vi "TestTabDisabled.vi"() -> ()   [LabVIEW 2022 SP3]
uses:
  Classes/TopLevel/Typedefs/PurgeMode--Enum.ctl
  Classes/TopLevel/Typedefs/AdvPrinterControl--Tabs.ctl
panel:
  in  "OK":bool
  in  "PrinterControls":T1
  out "ImageMain":T2(plugin-control)
  in  "Head6 Temp 1":string
  in  "Head5 Temp 1":string
  in  "Head4 Temp 1":string
  in  "Head3 Temp 1":string
  in  "Head2 Temp 1":string
  in  "Jog (+) 1":bool
  in  "Jog (-) 1":bool
  in  "Mode H1":T3
  in  "Mode H2":T3
  in  "Mode H3":T3
  in  "Mode H4":T3
  in  "Mode H5":T3
  in  "Mode H6":T3
  in  "Prime Repeats1 1":u8=1 min=1
  in  "Prime Repeats1 2":u8=1
  in  "Prime Repeats1 3":u8=1
  in  "Prime Repeats1 4":u8=1
  in  "Prime Repeats1 5":u8=1
  in  "Prime Repeats1 6":u8=1
  in  "StartPrime1 6":bool
  in  "StartPrime1 5":bool
  in  "StartPrime1 4":bool
  in  "StartPrime1 3":bool
  in  "StartPrime1 2":bool
  in  "StartPrime1 1":bool
  in  "Head1 Temp 1":string
  in  "Stage Head6":bool
  in  "Stage Head5":bool
  in  "Stage Head4":bool
  in  "Stage Head3":bool
  in  "Stage Head2":bool
  in  "Stage Head1":bool
  in  "Jog (+) 2":bool
  in  "Jog (-) 2":bool
  in  "Stage Recipe XML File Path":path
  in  "Start":bool
  in  "Stage Move Status":i32(listbox)
  in  "Idle Intervals (s)":dbl=0.1
  in  "IdlePrint":bool
  # "Jogging"
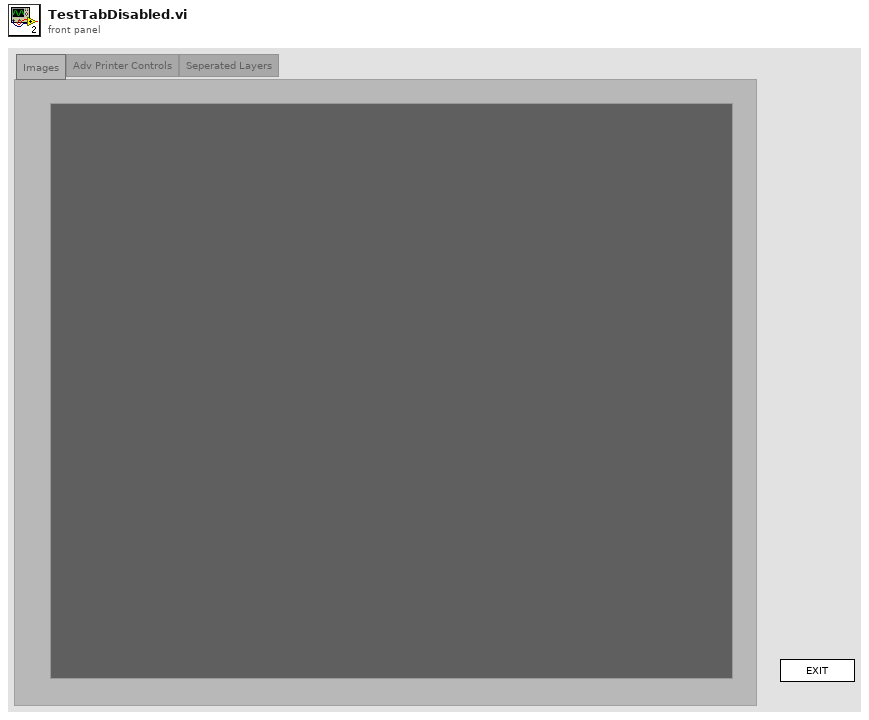
[diagram p1: front panel]
types:
  T1 = typedef "AdvPrinterControl--Tabs.ctl" = enum32{"Images", "Adv Printer Controls", "Seperated Layers"}
  T2 = typedef "IMAQ Image.ctl" = refnum<image>
  T3 = typedef "PurgeMode--Enum.ctl" = enum16{"Pre-Purge", "Purge", "Spit", "Prime"}
  T4 = enum8{"Enabled", "Disabled", "Disabled and Grayed Out"}
  T5 = enum32{"Invalid", "Standard", "Closed", "Hidden", "Minimized", "Maximized"}
  T6 = enum32{"invalid app kind", "Development System", "Run Time System", "Student Edition", "Embedded LabVIEW", "Evaluation", "Custom"}
  T7 = cluster{"Core":cluster{"Current VI Reference":refnum<vi>, "Close Panel on Exit?":bool}, "Your Boolean data":bool, "Your string data":string}
  T8 = cluster{"Current VI Reference":refnum<vi>, "Close Panel on Exit?":bool}
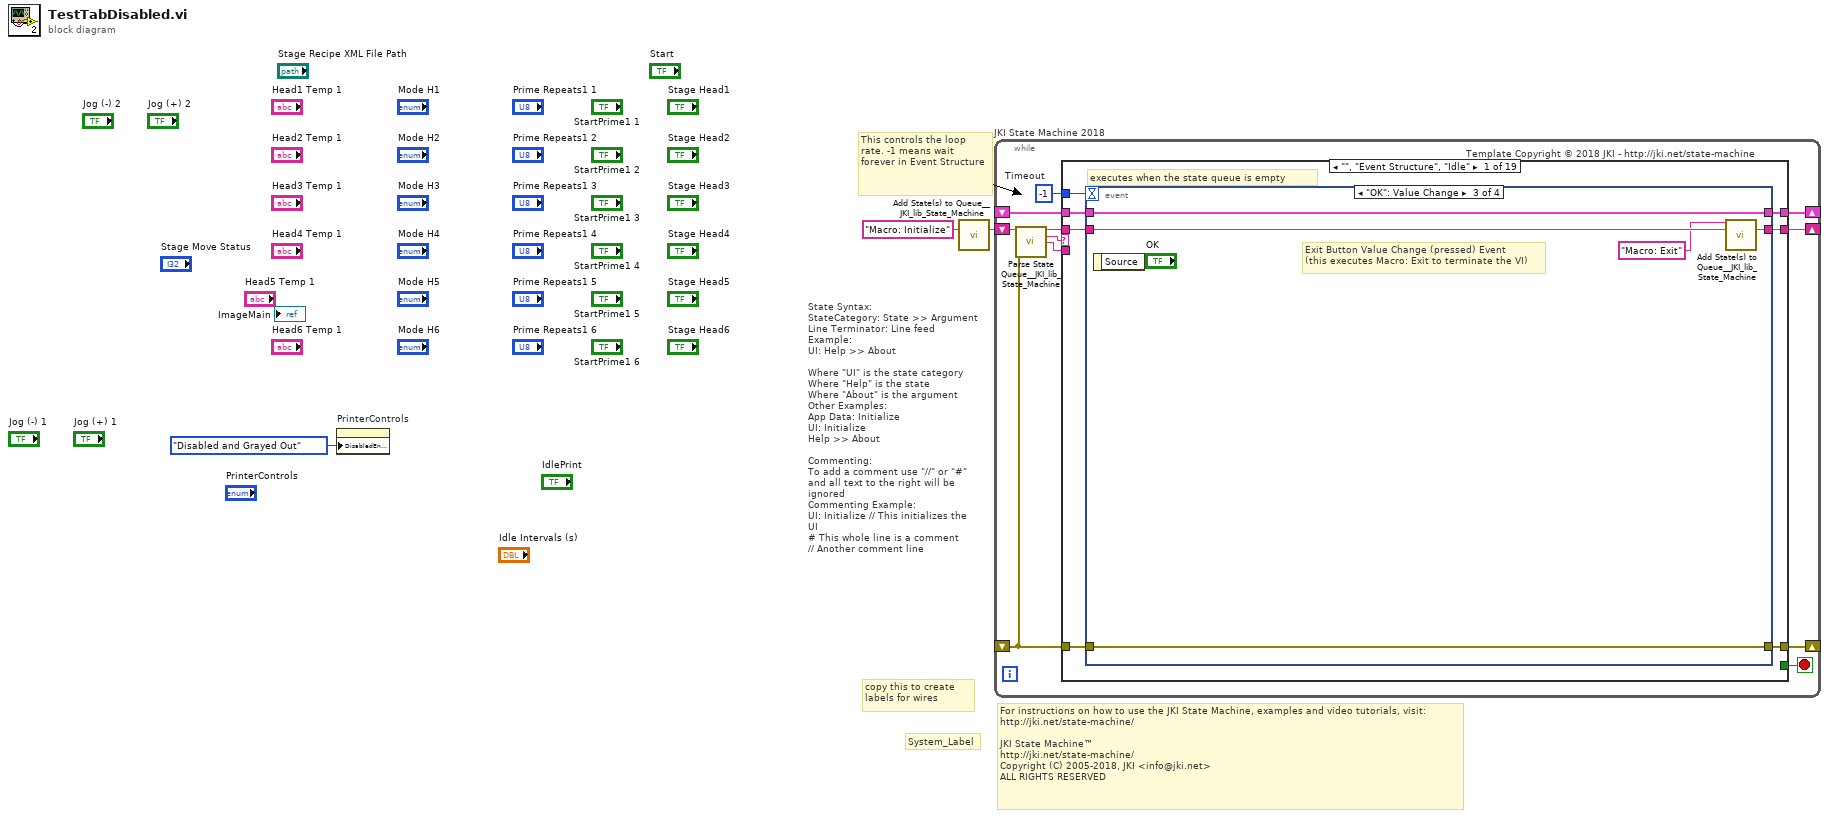
[diagram p0: block diagram]
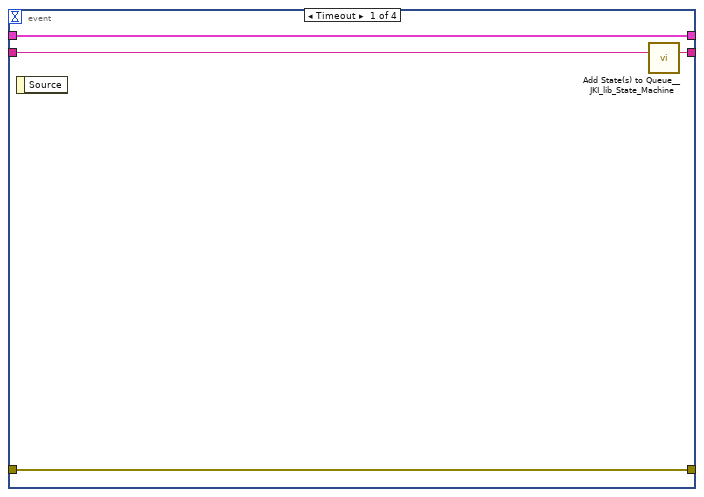
[diagram p2: hidden frame]
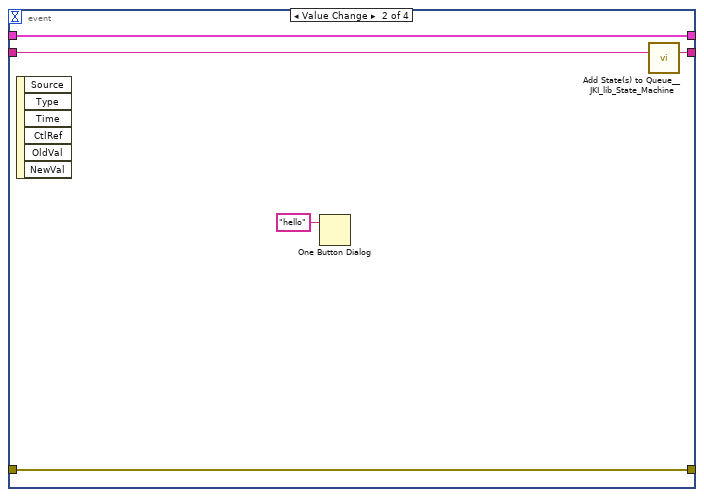
[diagram p3: hidden frame]
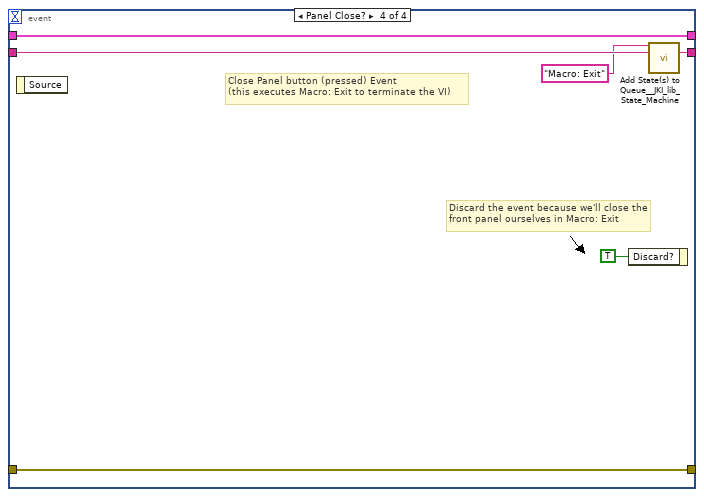
[diagram p4: hidden frame]
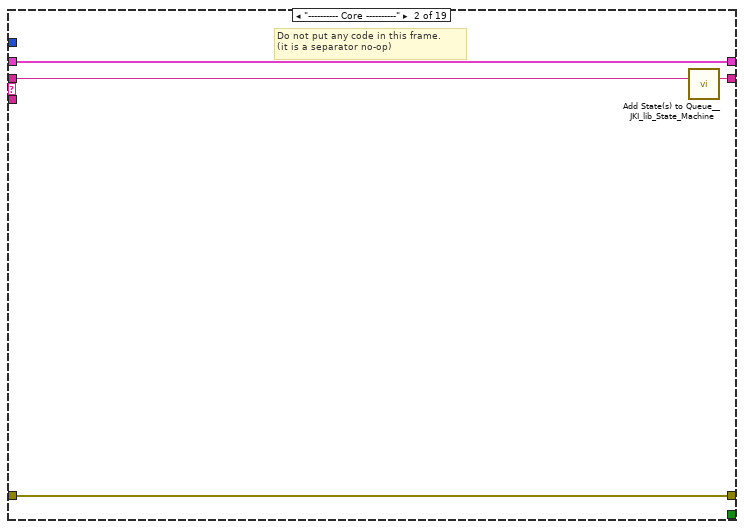
[diagram p5: hidden frame]
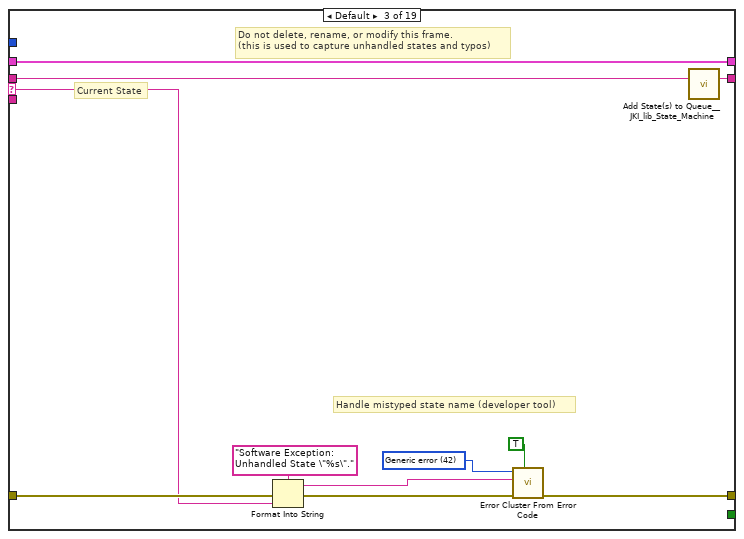
[diagram p6: hidden frame]
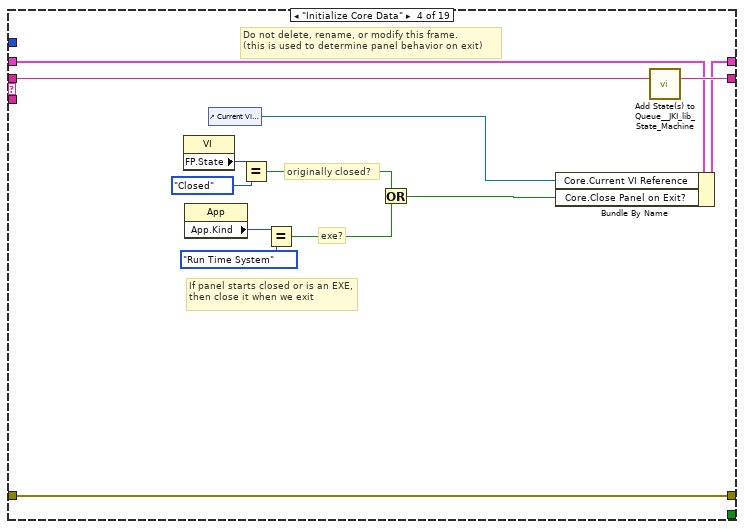
[diagram p7: hidden frame]
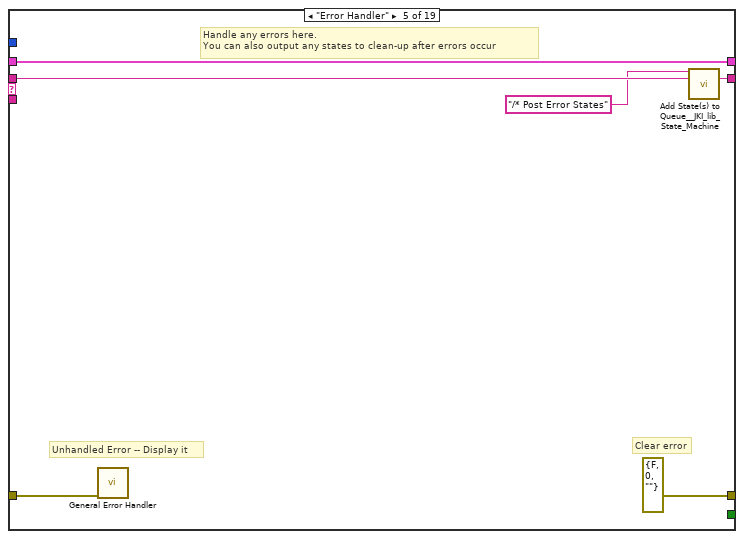
[diagram p8: hidden frame]
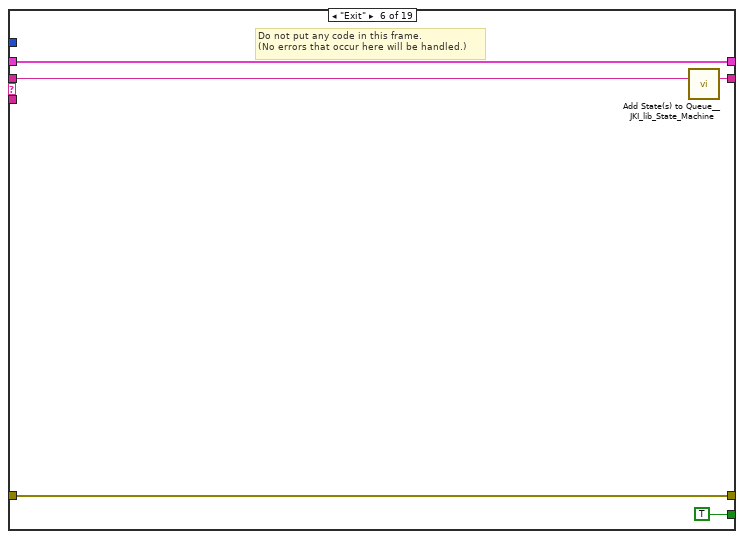
[diagram p9: hidden frame]
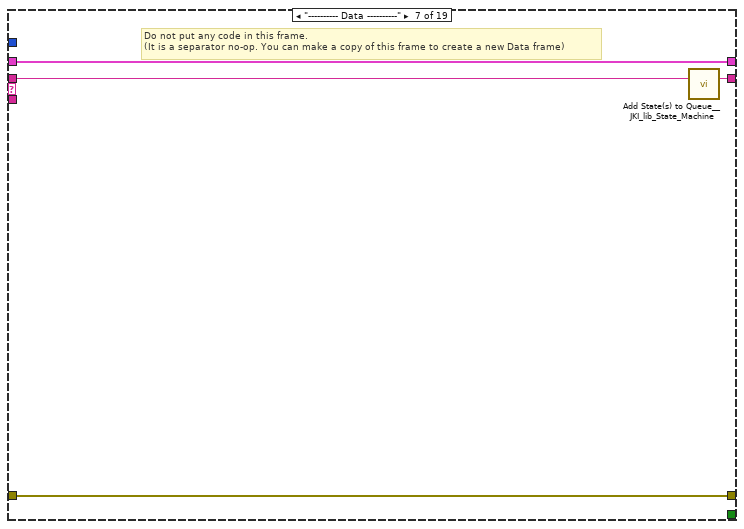
[diagram p10: hidden frame]
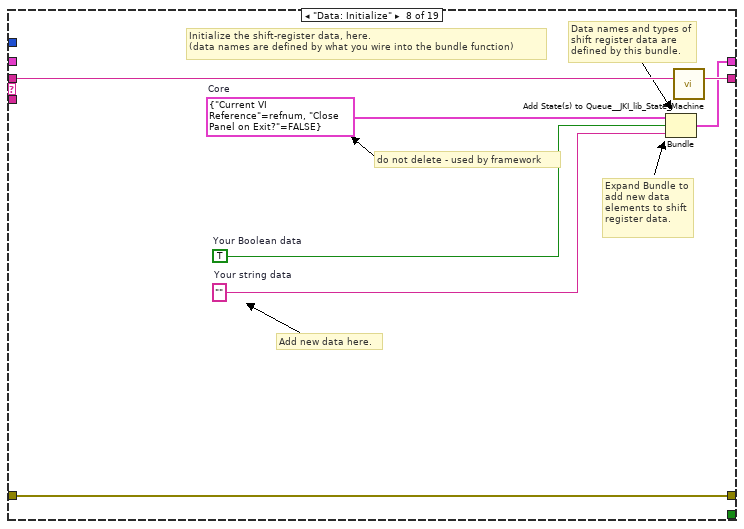
[diagram p11: hidden frame]
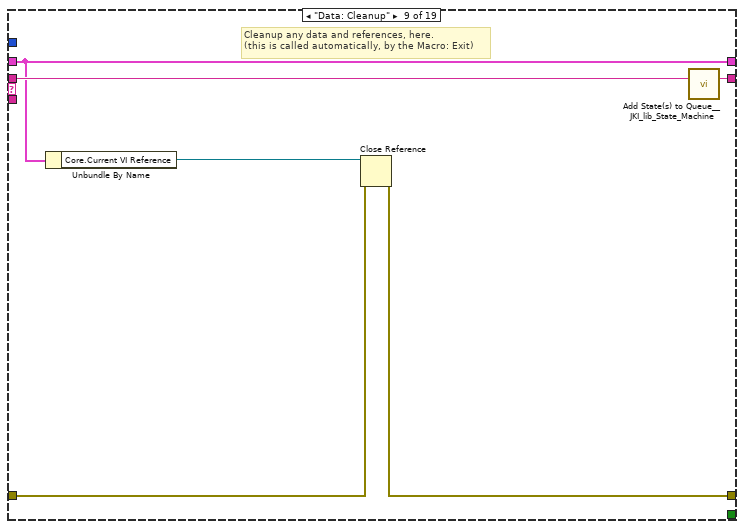
[diagram p12: hidden frame]
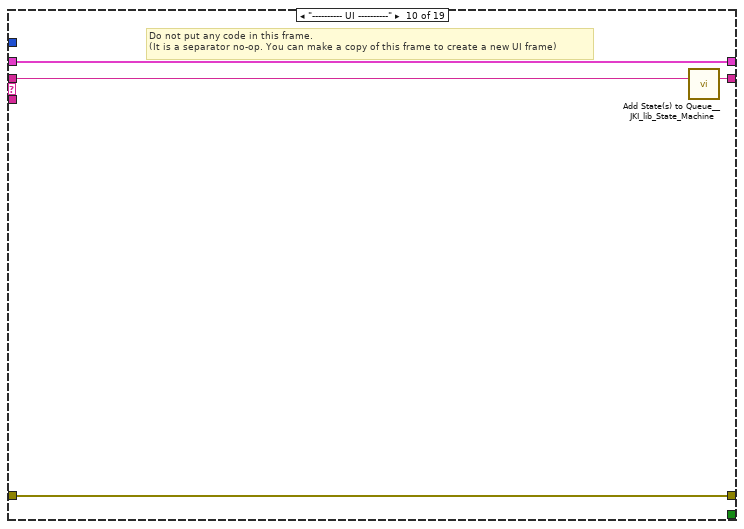
[diagram p13: hidden frame]
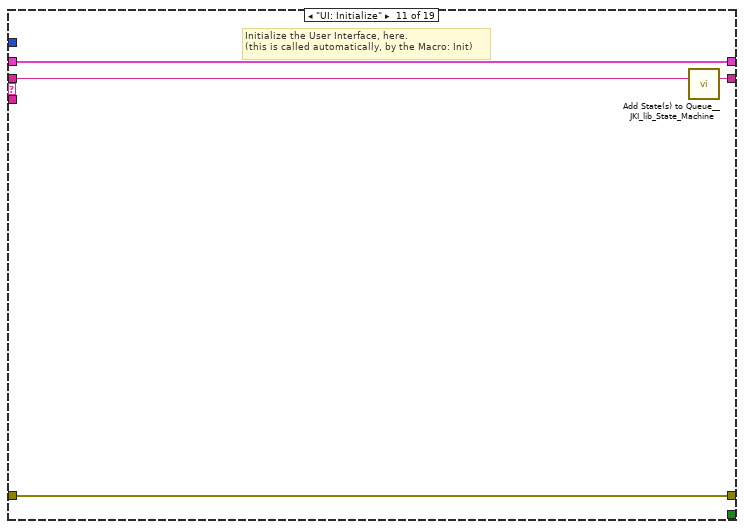
[diagram p14: hidden frame]
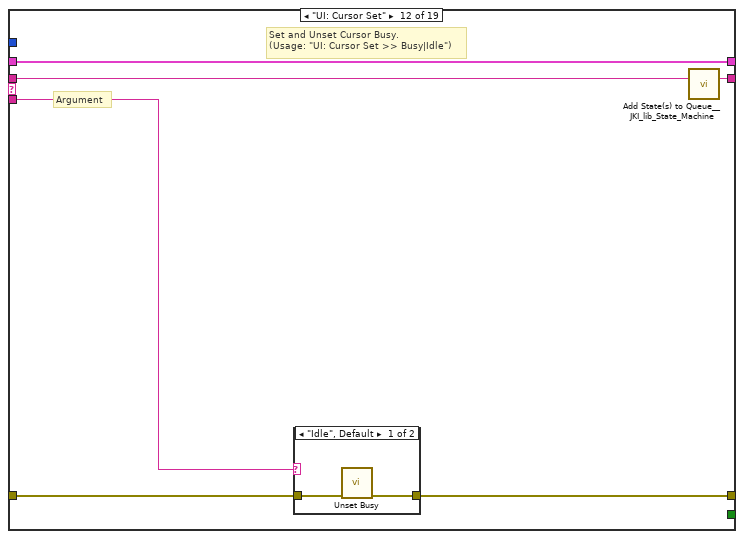
[diagram p15: hidden frame]
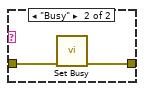
[diagram p16: hidden frame]
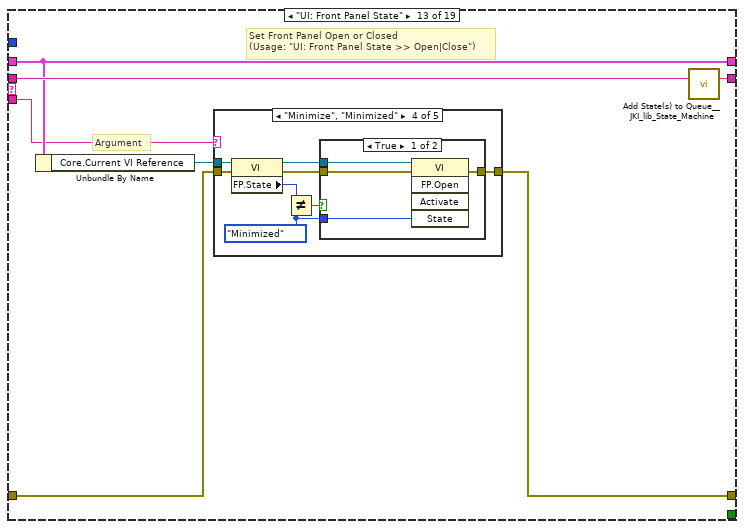
[diagram p17: hidden frame]
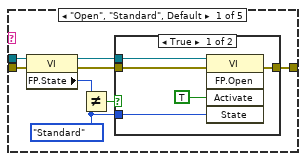
[diagram p18: hidden frame]
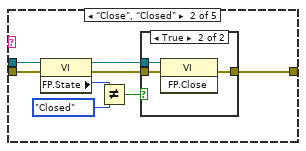
[diagram p20: hidden frame]
diagram:
  # "For instructions on how to use the JKI State Machine, examples and video tutorials, visit:\nhttp://jki.net/state-machine/\n\nJKI State Machine™\nhttp://jki.net/state-machine/\nCopyright (C) 2005-2018, JKI <info@jki.net>\nALL RIGHTS RESERVED"
  # "State Syntax:\nStateCategory: State >> Argument\nLine Terminator: Line feed\nExample:\nUI: Help >> About\n\nWhere \"UI\" is the state category\nWhere \"Help\" is the state\nWhere \"About\" is the argument\nOther Examples:\nApp Data: Initialize\nUI: Initialize\nHelp >> About\n\nCommenting:\nTo add a comment use \"//\" or \"#\" and all text to the right will be ignored\nCommenting Example:\nUI: Initialize // This initializes the UI\n# This whole line is a comment\n// Another comment line"
  # "copy this to create labels for wires"
  # "This controls the loop rate. -1 means wait forever in Event Structure"
  # "System_Label"
  n1 = property on="PrinterControls" class="TabCtl (strict)"("DisabledEnum"=T4."Disabled and Grayed Out" ("Disabled")) -> ()  [unwired: 2 in, 2 out]
  n2 = call <vilib>:"Add State(s) to Queue__JKI_lib_State_Machine.vi"("State(s) in (\"\")"="Macro: Initialize") -> ("States Out"=w2:string)  [unwired: 14 in]
  n3 = while "JKI State Machine 2018" {
    shift-right: [w7] -> _
    shift-left: _ -> [w6]
    shift-right: [w10] -> _
    shift-left: _ -> [w4]
    shift-right: [w9] -> _
    shift-left: w2 -> [w11]
    stop <- w8 stop-if-true
    w5 = -1  # Timeout
    # "Template Copyright © 2018 JKI - http://jki.net/state-machine"
    n4 = call <vilib>:"Parse State Queue__JKI_lib_State_Machine.vi"("State Queue"=w11, "Error In (no error)"=w4) -> ("Remaining States"=w13:string, "Current State"=w14:string, "Arguments"=w12:string)  [unwired: 11 in]
    n5 = case shown="\"\", \"Event Structure\", \"Idle\"" w14 {
      selector: w14 -> [_ _ w46 _ _ _ _ _ _ _ _ _ _ _ _ _ _ _ _]
      tunnel: w13 -> [w21 w45 w50 w69 w75 w80 w84 w91 w97 w101 w105 w111 w122 w191 w196 w206 w210 w214 w218]
      tunnel: w12 -> [_ _ _ _ _ _ _ _ _ _ _ w106 w116 _ _ _ _ _ _]
      tunnel: w6 -> [w19 w42 w48 w62 w72 w78 w81 _ w92 w98 w103 w109 w118 w188 w193 w203 w207 w211 w215]
      tunnel: [w18 w43 w52 w66 errorcluster {"status"=FALSE, "code"=0, "source"=""} ("error out") w77 w82 w88 w93 w99 w102 w107 w119 w189 w194 w204 w208 w212 w216] -> w10
      tunnel: w4 -> [w17 w43 w51 w66 w71 w77 w82 w88 w94 w99 w102 w108 w120 w189 w194 w204 w208 w212 w216]
      tunnel: [w20 w44 w49 w68 w74 w79 w83 w90 w96 w100 w104 w110 w121 w190 w195 w205 w209 w213 w217] -> w9
      tunnel: [_ _ _ _ _ TRUE _ _ _ _ _ _ _ _ _ _ _ _ _] -> w8
      tunnel: [w16 w42 w48 w67 w72 w78 w81 w89 w92 w98 w103 w109 w118 w188 w193 w203 w207 w211 w215] -> w7
      tunnel: w5 -> [w15 _ _ _ _ _ _ _ _ _ _ _ _ _ _ _ _ _ _]
      frame "", "Event Structure", "Idle" {
        # "executes when the state queue is empty"
        n6 = event shown="[2] \"OK\": Value Change" {
          selector: _ -> [_ _ _ _]
          dyn-events: _ -> [_ _ _ _]
          timeout: w15 -> [_ _ _ _]
          tunnel: w21 -> [w25 w30 w35 w41]
          tunnel: [w24 w29 w34 w40] -> w20
          tunnel: w19 -> [w22 w27 w32 w38]
          tunnel: [w23 w28 w33 w39] -> w18
          tunnel: w17 -> [w23 w28 w33 w39]
          tunnel: [w22 w27 w32 w38] -> w16
          event Timeout {
            n7 = event-data() -> ()  [unwired: 1 in, 1 out]
            n8 = call <vilib>:"Add State(s) to Queue__JKI_lib_State_Machine.vi"("State(s) in (\"\")"=w25) -> ("States Out"=w24:string)  [unwired: 14 in]
          }
          event Value Change {
            n9 = event-data() -> ()  [unwired: 1 in, 6 out]
            n10 = One Button Dialog(message="hello") -> ()  [unwired: 1 in, 1 out]
            n11 = call <vilib>:"Add State(s) to Queue__JKI_lib_State_Machine.vi"("State(s) in (\"\")"=w30) -> ("States Out"=w29:string)  [unwired: 14 in]
          }
          event "OK": Value Change {
            # "Exit Button Value Change (pressed) Event\n(this executes Macro: Exit to terminate the VI)"
            n12 = event-data() -> ()  [unwired: 1 in, 1 out]
            n13 = call <vilib>:"Add State(s) to Queue__JKI_lib_State_Machine.vi"("State(s) in Front (\"\")"="Macro: Exit", "State(s) in (\"\")"=w35) -> ("States Out"=w34:string)  [unwired: 13 in]
          }
          event Panel Close? {
            # "Discard the event because we'll close the front panel ourselves in Macro: Exit"
            # "Close Panel button (pressed) Event\n(this executes Macro: Exit to terminate the VI)"
            n14 = event-data() -> ()  [unwired: 1 in, 1 out]
            n15 = event-data("Discard?"=TRUE) -> ()  [unwired: 1 in, 1 out]
            n16 = call <vilib>:"Add State(s) to Queue__JKI_lib_State_Machine.vi"("State(s) in Front (\"\")"="Macro: Exit", "State(s) in (\"\")"=w41) -> ("States Out"=w40:string)  [unwired: 13 in]
          }
        }
      }
      frame "---------- Core ----------" {
        # "Do not put any code in this frame.\n(it is a separator no-op)"
        n17 = call <vilib>:"Add State(s) to Queue__JKI_lib_State_Machine.vi"("State(s) in (\"\")"=w45) -> ("States Out"=w44:string)  [unwired: 14 in]
      }
      frame Default {
        w55 = 42 items=["No error", "Argument error", "Memory is full", "Out of zone", "End of file", "File already open", "Generic file I/O error", "File not found", "File permission error", "Disk is full", "Duplicate path", "Too many files open", "System feature not enabled", "Resource file not found", "Cannot add resource", "Resource not found", "Image not found", "Image memory error", "Pen does not exist", "Config type invalid", "Config token not found", "Config parse error", "Config memory error", "Bad external code format", "Bad external code offset", "External code not present", "Null window", "Destroy window error", "Null menu", "Print aborted", "Bad print record", "Print driver error", "Windows error during printing", "Memory error during printing", "Print dialog error", "Generic print error", "Invalid device refnum", "Device not found", "Device parameter error", "Device unit error", "Cannot open device", "Device call aborted", "Generic error", "Cancelled by user", "Object ID too low", "Object ID too high", "Object not in heap", "Unknown heap", "Unknown object (invalid DefProc)", "Unknown object (DefProc not in table)", "Message out of range", "Invalid (null) method", "Unknown message", "Manager call not supported", "Bad address", "Network operation in progress", "Network operation timed out", "Connection is busy", "Network attribute not supported", "Network error", "Address in use", "System out of memory", "Connection aborted", "Connection refused", "Not connected", "Already connected", "Connection closed", "Initialization error (interapplication manager)", "Bad occurrence", "Wait on unbound occurrence handler", "Occurrence queue overflow", "Datalog type conflict", "Unused", "Unrecognized type (interapplication manager)", "Memory corrupt", "Failed to make temporary DLL", "Old CIN version", "Drag socket not found", "Failed to load drop-object", "Failed to register OLE object", "Failed to release OLE object", "Format specifier type mismatch", "Unknown format specifier", "Too few format specifiers", "Too many format specifiers", "Scan failed", "Newer CIN version", "Error converting to variant", "Runtime menu error", "Password tampered", "Variant attribute not found", "Incompatible variant data type", "Event data is not available", "Event Store is not present", "Occurrence is not found", "Event Queue is not created", "Event info is not available", "Refnum passed is NULL", "Error retrieving Class GUID", "Error retrieving CoClass GUID", "Error retrieving TypeLib GUID.", "Bad built application magic bytes.", "Specific driver is different from the specific driver associated with the Logical Name.", "There is no session opened to the class driver.", "Max Error", "MAX - Error with config objects", "MAX - Error loading configuration", "MAX - Group not supported"]
        # "Current State"
        # "Do not delete, rename, or modify this frame.\n(this is used to capture unhandled states and typos)"
        # "Handle mistyped state name (developer tool)"
        n18 = Format Into String(format string="Software Exception: Unhandled State \"%s\"." ("message"), error in=w51, w46) -> (resulting string=w54:string, error out=w53:errorcluster)  [unwired: 1 in]
        n19 = call <vilib>:"Error Cluster From Error Code.vi"("show call chain? (False)"=TRUE, "error in (no error)"=w53, "error message (\"\")"=w54, "error code (0)"=w55) -> ("error out"=w52:errorcluster)  [unwired: 5 in]
        n20 = call <vilib>:"Add State(s) to Queue__JKI_lib_State_Machine.vi"("State(s) in (\"\")"=w50) -> ("States Out"=w49:string)  [unwired: 14 in]
      }
      frame "Initialize Core Data" {
        # "Do not delete, rename, or modify this frame.\n(this is used to determine panel behavior on exit)"
        # "originally closed?"
        # "exe?"
        # "If panel starts closed or is an EXE, then close it when we exit"
        n21 = property class="VI"() -> ("FP.State"=w59:T5)  [unwired: 2 in, 2 out]
        n22 = property class="App"() -> ("App.Kind"=w65:T6)  [unwired: 2 in, 2 out]
        n23 = control-ref of="Current VI Reference"() -> (w60:refnum<vi>)
        n24 = Equal?(x=w59, y=T5."Closed" ("Front Panel Window:State")) -> (x = y?=w57:bool)
        n25 = Equal?(x=w65, y=T6."Run Time System" ("Application:Kind")) -> (x = y?=w63:bool)
        n26 = Or(x=w57, y=w63) -> (x .or. y?=w61:bool)
        n27 = Bundle By Name(cluster=w62, "Core.Current VI Reference"=w60, "Core.Close Panel on Exit?"=w61) -> (w67:T7)
        n28 = call <vilib>:"Add State(s) to Queue__JKI_lib_State_Machine.vi"("State(s) in (\"\")"=w69) -> ("States Out"=w68:string)  [unwired: 14 in]
      }
      frame "Error Handler" {
        # "Unhandled Error -- Display it"
        # "Handle any errors here.\nYou can also output any states to clean-up after errors occur"
        # "Clear error"
        n29 = call <vilib>:"General Error Handler.vi"("error in (no error)"=w71) -> ()  [unwired: 10 in, 5 out]
        n30 = call <vilib>:"Add State(s) to Queue__JKI_lib_State_Machine.vi"("State(s) in Front (\"\")"="/* Post Error States", "State(s) in (\"\")"=w75) -> ("States Out"=w74:string)  [unwired: 13 in]
      }
      frame "Exit" {
        # "Do not put any code in this frame.\n(No errors that occur here will be handled.)"
        n31 = call <vilib>:"Add State(s) to Queue__JKI_lib_State_Machine.vi"("State(s) in (\"\")"=w80) -> ("States Out"=w79:string)  [unwired: 14 in]
      }
      frame "---------- Data ----------" {
        # "Do not put any code in this frame.\n(It is a separator no-op. You can make a copy of this frame to create a new Data frame)"
        n32 = call <vilib>:"Add State(s) to Queue__JKI_lib_State_Machine.vi"("State(s) in (\"\")"=w84) -> ("States Out"=w83:string)  [unwired: 14 in]
      }
      frame "Data: Initialize" {
        w85 = T8 {"Current VI Reference"=refnum, "Close Panel on Exit?"=FALSE}  # Core
        w87 = TRUE  # Your Boolean data
        w86 = ""  # Your string data
        # "do not delete - used by framework"
        # "Expand Bundle to add new data elements to shift register data."
        # "Add new data here."
        # "Data names and types of shift register data are defined by this bundle."
        # "Initialize the shift-register data, here.\n(data names are defined by what you wire into the bundle function)"
        n33 = Bundle("Core"=w85, "Your Boolean data"=w87, "Your string data"=w86) -> (w89:T7)  [unwired: 1 in]
        n34 = call <vilib>:"Add State(s) to Queue__JKI_lib_State_Machine.vi"("State(s) in (\"\")"=w91) -> ("States Out"=w90:string)  [unwired: 14 in]
      }
      frame "Data: Cleanup" {
        # "Cleanup any data and references, here.\n(this is called automatically, by the Macro: Exit)"
        n35 = Unbundle By Name(w92) -> ("Core.Current VI Reference"=w95:refnum<vi>)
        n36 = Close Reference(reference=w95, error in (no error)=w94) -> (error out=w93:errorcluster)
        n37 = call <vilib>:"Add State(s) to Queue__JKI_lib_State_Machine.vi"("State(s) in (\"\")"=w97) -> ("States Out"=w96:string)  [unwired: 14 in]
      }
      frame "---------- UI ----------" {
        # "Do not put any code in this frame.\n(It is a separator no-op. You can make a copy of this frame to create a new UI frame)"
        n38 = call <vilib>:"Add State(s) to Queue__JKI_lib_State_Machine.vi"("State(s) in (\"\")"=w101) -> ("States Out"=w100:string)  [unwired: 14 in]
      }
      frame "UI: Initialize" {
        # "Initialize the User Interface, here.\n(this is called automatically, by the Macro: Init)"
        n39 = call <vilib>:"Add State(s) to Queue__JKI_lib_State_Machine.vi"("State(s) in (\"\")"=w105) -> ("States Out"=w104:string)  [unwired: 14 in]
      }
      frame "UI: Cursor Set" {
        # "Argument"
        # "Set and Unset Cursor Busy.\n(Usage: \"UI: Cursor Set >> Busy|Idle\")"
        n40 = case shown="\"Idle\", Default" w106 {
          tunnel: w108 -> [w113 w115]
          tunnel: [w112 w114] -> w107
          frame "Idle", Default {
            n41 = call <vilib>:"Unset Busy.vi"("error in (no error)"=w113) -> ("error out"=w112:errorcluster)  [unwired: 10 in]
          }
          frame "Busy" {
            n42 = call <vilib>:"Set Busy.vi"("error in (no error)"=w115) -> ("error out"=w114:errorcluster)  [unwired: 9 in, 1 out]
          }
        }
        n43 = call <vilib>:"Add State(s) to Queue__JKI_lib_State_Machine.vi"("State(s) in (\"\")"=w111) -> ("States Out"=w110:string)  [unwired: 14 in]
      }
      frame "UI: Front Panel State" {
        # "Argument"
        # "Set Front Panel Open or Closed\n(Usage: \"UI: Front Panel State >> Open|Close\")"
        n44 = Unbundle By Name(w118) -> ("Core.Current VI Reference"=w117:refnum<vi>)
        n45 = case shown="\"Minimize\", \"Minimized\"" w116 {
          tunnel: w120 -> [w128 w143 w154 w167 w180]
          tunnel: [w130 w144 w156 w169 w182] -> w119
          tunnel: w117 -> [w129 w141 w155 w168 w181]
          frame "Open", "Standard", Default {
            w123 = T5."Standard" ("State")
            n46 = property class="VI"(reference=w129, error in=w128) -> (reference out=w126:refnum<vi>, error out=w127:errorcluster, "FP.State"=w125:T5)
            n47 = Not Equal?(x=w125, y=w123) -> (x != y?=w124:bool)
            n48 = case shown="True" w124 {
              tunnel: [w134 w136] -> w130
              tunnel: w127 -> [w133 w136]
              tunnel: w126 -> [w132 _]
              tunnel: w123 -> [w131 _]
              frame True {
                n49 = invoke class="VI" method="FP.Open"(reference=w132, error in=w133, "Activate"=TRUE, "State"=w131) -> (error out=w134:errorcluster)  [unwired: 1 in, 4 out]
              }
              frame False {
              }
            }
          }
          frame "Close", "Closed" {
            n50 = property class="VI"(reference=w141, error in=w143) -> (reference out=w140:refnum<vi>, error out=w142:errorcluster, "FP.State"=w138:T5)
            n51 = Not Equal?(x=w138, y=T5."Closed" ("Front Panel Window:State")) -> (x != y?=w137:bool)
            n52 = case shown="True" w137 {
              tunnel: [w145 w148] -> w144
              tunnel: w142 -> [w145 w147]
              tunnel: w140 -> [_ w146]
              frame False {
              }
              frame True {
                n53 = invoke class="VI" method="FP.Close"(reference=w146, error in=w147) -> (error out=w148:errorcluster)  [unwired: 1 in, 2 out]
              }
            }
          }
          frame "Hidden", "Hide" {
            w149 = T5."Hidden" ("State")
            n54 = property class="VI"(reference=w155, error in=w154) -> (reference out=w152:refnum<vi>, error out=w153:errorcluster, "FP.State"=w151:T5)
            n55 = Not Equal?(x=w151, y=w149) -> (x != y?=w150:bool)
            n56 = case shown="True" w150 {
              tunnel: [w160 w161] -> w156
              tunnel: w153 -> [w159 w161]
              tunnel: w152 -> [w158 _]
              tunnel: w149 -> [w157 _]
              frame True {
                n57 = invoke class="VI" method="FP.Open"(reference=w158, error in=w159, "State"=w157) -> (error out=w160:errorcluster)  [unwired: 2 in, 4 out]
              }
              frame False {
              }
            }
          }
          frame "Minimize", "Minimized" {
            w162 = T5."Minimized" ("State")
            n58 = property class="VI"(reference=w168, error in=w167) -> (reference out=w165:refnum<vi>, error out=w166:errorcluster, "FP.State"=w164:T5)
            n59 = Not Equal?(x=w164, y=w162) -> (x != y?=w163:bool)
            n60 = case shown="True" w163 {
              tunnel: [w173 w174] -> w169
              tunnel: w166 -> [w172 w174]
              tunnel: w165 -> [w171 _]
              tunnel: w162 -> [w170 _]
              frame True {
                n61 = invoke class="VI" method="FP.Open"(reference=w171, error in=w172, "State"=w170) -> (error out=w173:errorcluster)  [unwired: 2 in, 4 out]
              }
              frame False {
              }
            }
          }
          frame "Maximize", "Maximized" {
            w175 = T5."Maximized" ("State")
            n62 = property class="VI"(reference=w181, error in=w180) -> (reference out=w178:refnum<vi>, error out=w179:errorcluster, "FP.State"=w177:T5)
            n63 = Not Equal?(x=w177, y=w175) -> (x != y?=w176:bool)
            n64 = case shown="True" w176 {
              tunnel: [w186 w187] -> w182
              tunnel: w179 -> [w185 w187]
              tunnel: w178 -> [w184 _]
              tunnel: w175 -> [w183 _]
              frame True {
                n65 = invoke class="VI" method="FP.Open"(reference=w184, error in=w185, "State"=w183) -> (error out=w186:errorcluster)  [unwired: 2 in, 4 out]
              }
              frame False {
              }
            }
          }
        }
        n66 = call <vilib>:"Add State(s) to Queue__JKI_lib_State_Machine.vi"("State(s) in (\"\")"=w122) -> ("States Out"=w121:string)  [unwired: 14 in]
      }
      frame "---------- Macro ----------" {
        # "Do not put any code in this frame.\n(It is a separator no-op. You can make a copy of this frame to create a new Macro frame)"
        n67 = call <vilib>:"Add State(s) to Queue__JKI_lib_State_Machine.vi"("State(s) in (\"\")"=w191) -> ("States Out"=w190:string)  [unwired: 14 in]
      }
      frame "Macro: Initialize" {
        w192 = "Data: Initialize\nInitialize Core Data\nUI: Initialize\nUI: Front Panel State >> Open"  # Data: Initialize Initialize Core Data UI: Initialize UI: Front Panel State >> Open
        # "Initialization Macro\n(This is called once, when the VI starts)"
        n68 = call <vilib>:"Add State(s) to Queue__JKI_lib_State_Machine.vi"("State(s) in Front (\"\")"=w192, "State(s) in (\"\")"=w196) -> ("States Out"=w195:string)  [unwired: 13 in]
      }
      frame "Macro: Exit" {
        # "Exit Macro\n(This is called once, when the VI exits)"
        n69 = Unbundle By Name(w203) -> ("Core.Close Panel on Exit?"=w202:bool)
        n70 = Select(t="UI: Front Panel State >> Close", s=w202, f="") -> (s? t:f=w199:string)
        n71 = call <vilib>:"Add State(s) to Queue__JKI_lib_State_Machine.vi"("State(s) in (\"\")"=w199, "State(s) at Back (\"\")"="Data: Cleanup\nExit") -> ("States Out"=w197:string)  [unwired: 13 in]
        n72 = call <vilib>:"Add State(s) to Queue__JKI_lib_State_Machine.vi"("State(s) in Front (\"\")"=w197, "State(s) in (\"\")"=w206) -> ("States Out"=w205:string)  [unwired: 13 in]
      }
      frame "---------- New Category ----------" {
        # "Template Separator\n(You can make a copy of, or modify, this frame)"
        n73 = call <vilib>:"Add State(s) to Queue__JKI_lib_State_Machine.vi"("State(s) in (\"\")"=w210) -> ("States Out"=w209:string)  [unwired: 14 in]
      }
      frame "New Category: 1" {
        # "Your code here.\n(You can make a copy of, or modify, this frame)"
        n74 = call <vilib>:"Add State(s) to Queue__JKI_lib_State_Machine.vi"("State(s) in (\"\")"=w214) -> ("States Out"=w213:string)  [unwired: 14 in]
      }
      frame "New Category: 2" {
        # "Your code here.\n(You can make a copy of, or modify, this frame)"
        n75 = call <vilib>:"Add State(s) to Queue__JKI_lib_State_Machine.vi"("State(s) in (\"\")"=w218) -> ("States Out"=w217:string)  [unwired: 14 in]
      }
    }
  }
